vi "Read String.vi"(11 "Event in":refnum<class "Event String.lvclass">) -> (2 "String":string, 3 "Event out":refnum<class "Event String.lvclass">)   [LabVIEW 2016, in "Event Source.lvlib" / "Event String.lvclass"]
uses:
  Event String.lvclass
  Event String.lvclass/Event String.ctl
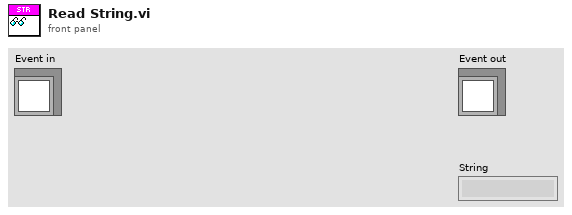
[diagram p1: front panel]
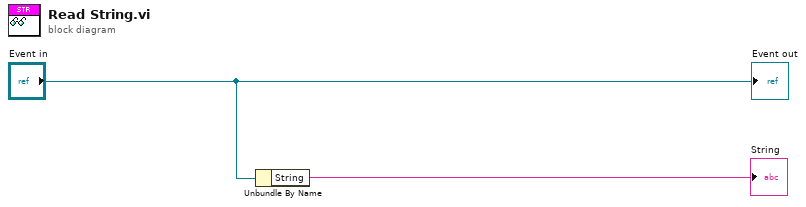
[diagram p0: block diagram]
diagram:
  n1 = Unbundle By Name("Event in") -> ("String"=→"String":string)
  "Event out" <- "Event in"
